vi "Is2DArray.vi"(3 "Datatype":T1, 4 "Value String in":string) -> (0 "IsArray":bool, 2 "Array Value":variant)   [LabVIEW 2016]
uses:
  Datatype.ctl
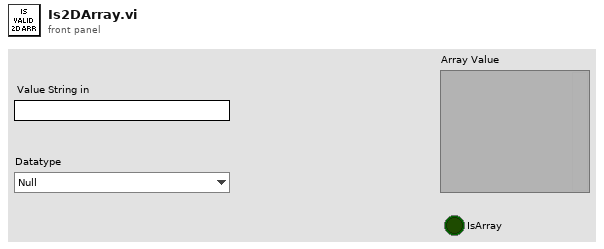
[diagram p1: front panel]
types:
  T1 = typedef "Datatype.ctl" = enum16{"Null", "Numeric", "String", "Bool", "Numeric 1D", "String 1D", "Bool 1D", "Numeric 2D", "String 2D", "Bool 2D", "Variant"}
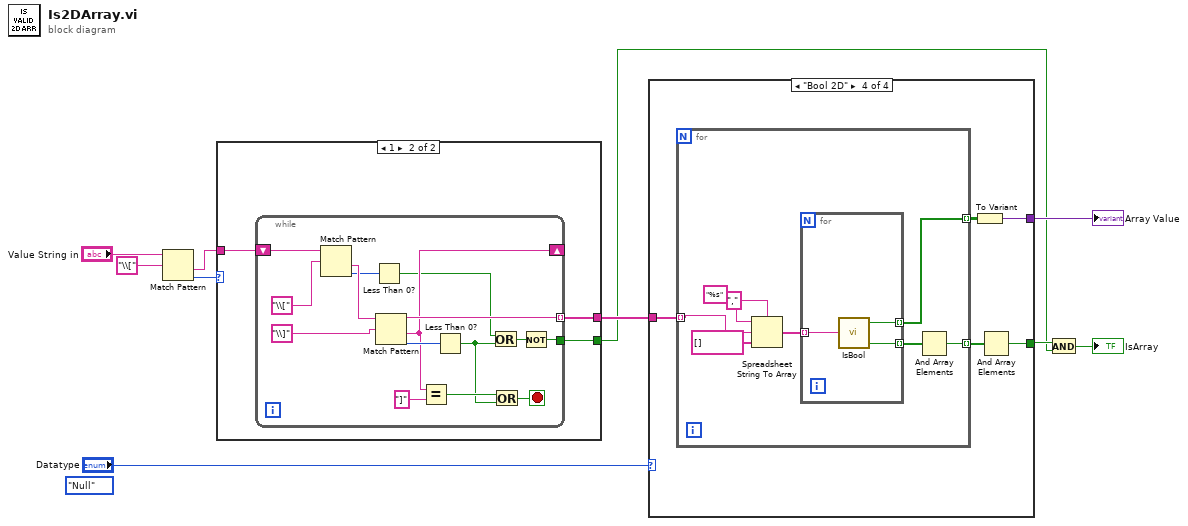
[diagram p0: block diagram]
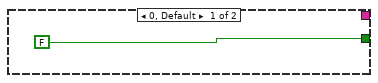
[diagram p2: hidden frame]
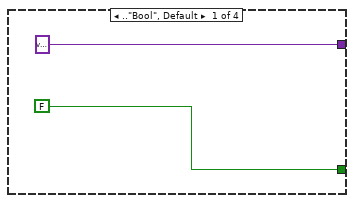
[diagram p3: hidden frame]
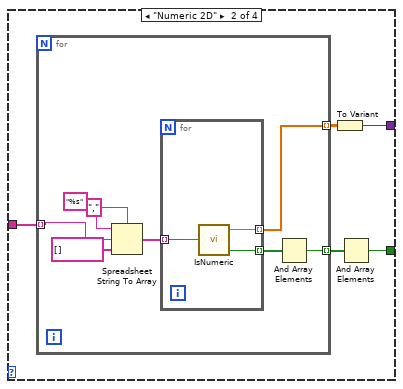
[diagram p4: hidden frame]
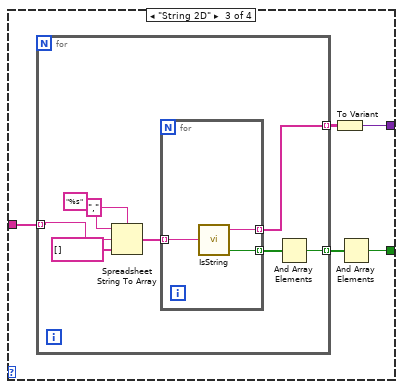
[diagram p5: hidden frame]
diagram:
  (unwired) Datatype."Null" ("Datatype")
  n1 = Match Pattern(string="Value String in", regular expression="\\[") -> (after substring=w5:string, offset past match=w6:i32)  [unwired: 1 in, 2 out]
  n2 = case shown="1" w6 {
    tunnel: w5 -> [_ w14]
    tunnel: [_ w13] -> w4
    tunnel: [FALSE w12] -> w1
    frame 0, Default {
    }
    frame 1 {
      n3 = while {
        tunnel: [w25] -> w13 mode=indexing
        shift-right: [w20] -> _
        shift-left: w14 -> [w28]
        tunnel: [w15] -> w12
        stop <- w22 stop-if-true
        n4 = Match Pattern(string=w28, regular expression="\\[") -> (after substring=w27:string, offset past match=w18:i32)  [unwired: 1 in, 2 out]
        n5 = Less Than 0?(x=w18) -> (x < 0?=w16:bool)
        n6 = Match Pattern(string=w27, regular expression="\\]") -> (before substring=w25:string, after substring=w20:string, offset past match=w21:i32)  [unwired: 1 in, 1 out]
        n7 = Equal?(x=w20, y="]") -> (x = y?=w24:bool)
        n8 = Less Than 0?(x=w21) -> (x < 0?=w19:bool)
        n9 = Or(x=w16, y=w19) -> (x .or. y?=w17:bool)
        n10 = Or(x=w24, y=w19) -> (x .or. y?=w22:bool)
        n11 = Not(x=w17) -> (.not. x?=w15:bool)
      }
    }
  }
  n12 = case shown="\"Bool 2D\"" "Datatype" {
    tunnel: [FALSE w32 w48 w64] -> w3
    tunnel: [variant w34 w50 w66] -> w9
    tunnel: w4 -> [_ w35 w51 w67]
    frame .."Bool", Default {
    }
    frame "Numeric 2D" {
      n13 = for {
        tunnel: [w39] -> w33 mode=indexing
        tunnel: [w37] -> w36 mode=indexing
        tunnel: w35 -> [w38] mode=indexing
        n14 = Spreadsheet String To Array(delimiter (Tab)=",", format string="%s", spreadsheet string=w38, array type (2D Dbl)=string[] []) -> (array=w41:string[])
        n15 = for {
          tunnel: w41 -> [w47] mode=indexing
          tunnel: [w46] -> w37 mode=indexing
          tunnel: [w45] -> w40 mode=indexing
          n16 = call "IsNumeric.vi"("Value String in"=w47) -> ("IsNumeric"=w45:bool, "Numeric Value"=w46:ext)  [unwired: 3 in]
        }
        n17 = And Array Elements(Boolean array=w40) -> (logical AND=w39:bool)
      }
      n18 = To Variant(anything=w36) -> (Variant=w34:variant)
      n19 = And Array Elements(Boolean array=w33) -> (logical AND=w32:bool)
    }
    frame "String 2D" {
      n20 = for {
        tunnel: [w55] -> w49 mode=indexing
        tunnel: [w53] -> w52 mode=indexing
        tunnel: w51 -> [w54] mode=indexing
        n21 = Spreadsheet String To Array(delimiter (Tab)=",", format string="%s", spreadsheet string=w54, array type (2D Dbl)=string[] []) -> (array=w57:string[])
        n22 = for {
          tunnel: w57 -> [w63] mode=indexing
          tunnel: [w62] -> w53 mode=indexing
          tunnel: [w61] -> w56 mode=indexing
          n23 = call "IsString.vi"("Value String in"=w63) -> ("IsString"=w61:bool, "String Value"=w62:string)  [unwired: 3 in]
        }
        n24 = And Array Elements(Boolean array=w56) -> (logical AND=w55:bool)
      }
      n25 = To Variant(anything=w52) -> (Variant=w50:variant)
      n26 = And Array Elements(Boolean array=w49) -> (logical AND=w48:bool)
    }
    frame "Bool 2D" {
      n27 = for {
        tunnel: [w71] -> w65 mode=indexing
        tunnel: [w69] -> w68 mode=indexing
        tunnel: w67 -> [w70] mode=indexing
        n28 = Spreadsheet String To Array(delimiter (Tab)=",", format string="%s", spreadsheet string=w70, array type (2D Dbl)=string[] []) -> (array=w73:string[])
        n29 = for {
          tunnel: w73 -> [w79] mode=indexing
          tunnel: [w78] -> w69 mode=indexing
          tunnel: [w77] -> w72 mode=indexing
          n30 = call "IsBool.vi"("Value String in"=w79) -> ("IsBool"=w77:bool, "Bool Value"=w78:bool)  [unwired: 3 in]
        }
        n31 = And Array Elements(Boolean array=w72) -> (logical AND=w71:bool)
      }
      n32 = To Variant(anything=w68) -> (Variant=w66:variant)
      n33 = And Array Elements(Boolean array=w65) -> (logical AND=w64:bool)
    }
  }
  "Array Value" <- w9
  n34 = And(x=w3, y=w1) -> (x .and. y?=→"IsArray":bool)
